vi "Main Test.vi"() -> ()   [LabVIEW 2021]
uses:
  Mete.ctl
  R.ctl
  P.ctl
  N.ctl
  D.ctl
  Odo Velocity.ctl
  Gas.ctl
  Set-.ctl
  Set+.ctl
  Cru.ctl
  Dis.ctl
panel:
  in  "Boolean 8":T1
  in  "Boolean 7":T2
  in  "Boolean 5":T3
  in  "Boolean 6":T4
  in  "Slide 2":T5
  out "Km/h":T6 scale=0.0..250.0
  in  "stop":bool
  in  "Slide":u32(slide) max=900 scale=0.0..999.0
  out "Boolean 4":T7
  out "Boolean 3":T8
  out "Boolean 2":T9
  out "Boolean":T10
  out "Gauge":T11 scale=0.0..650.0
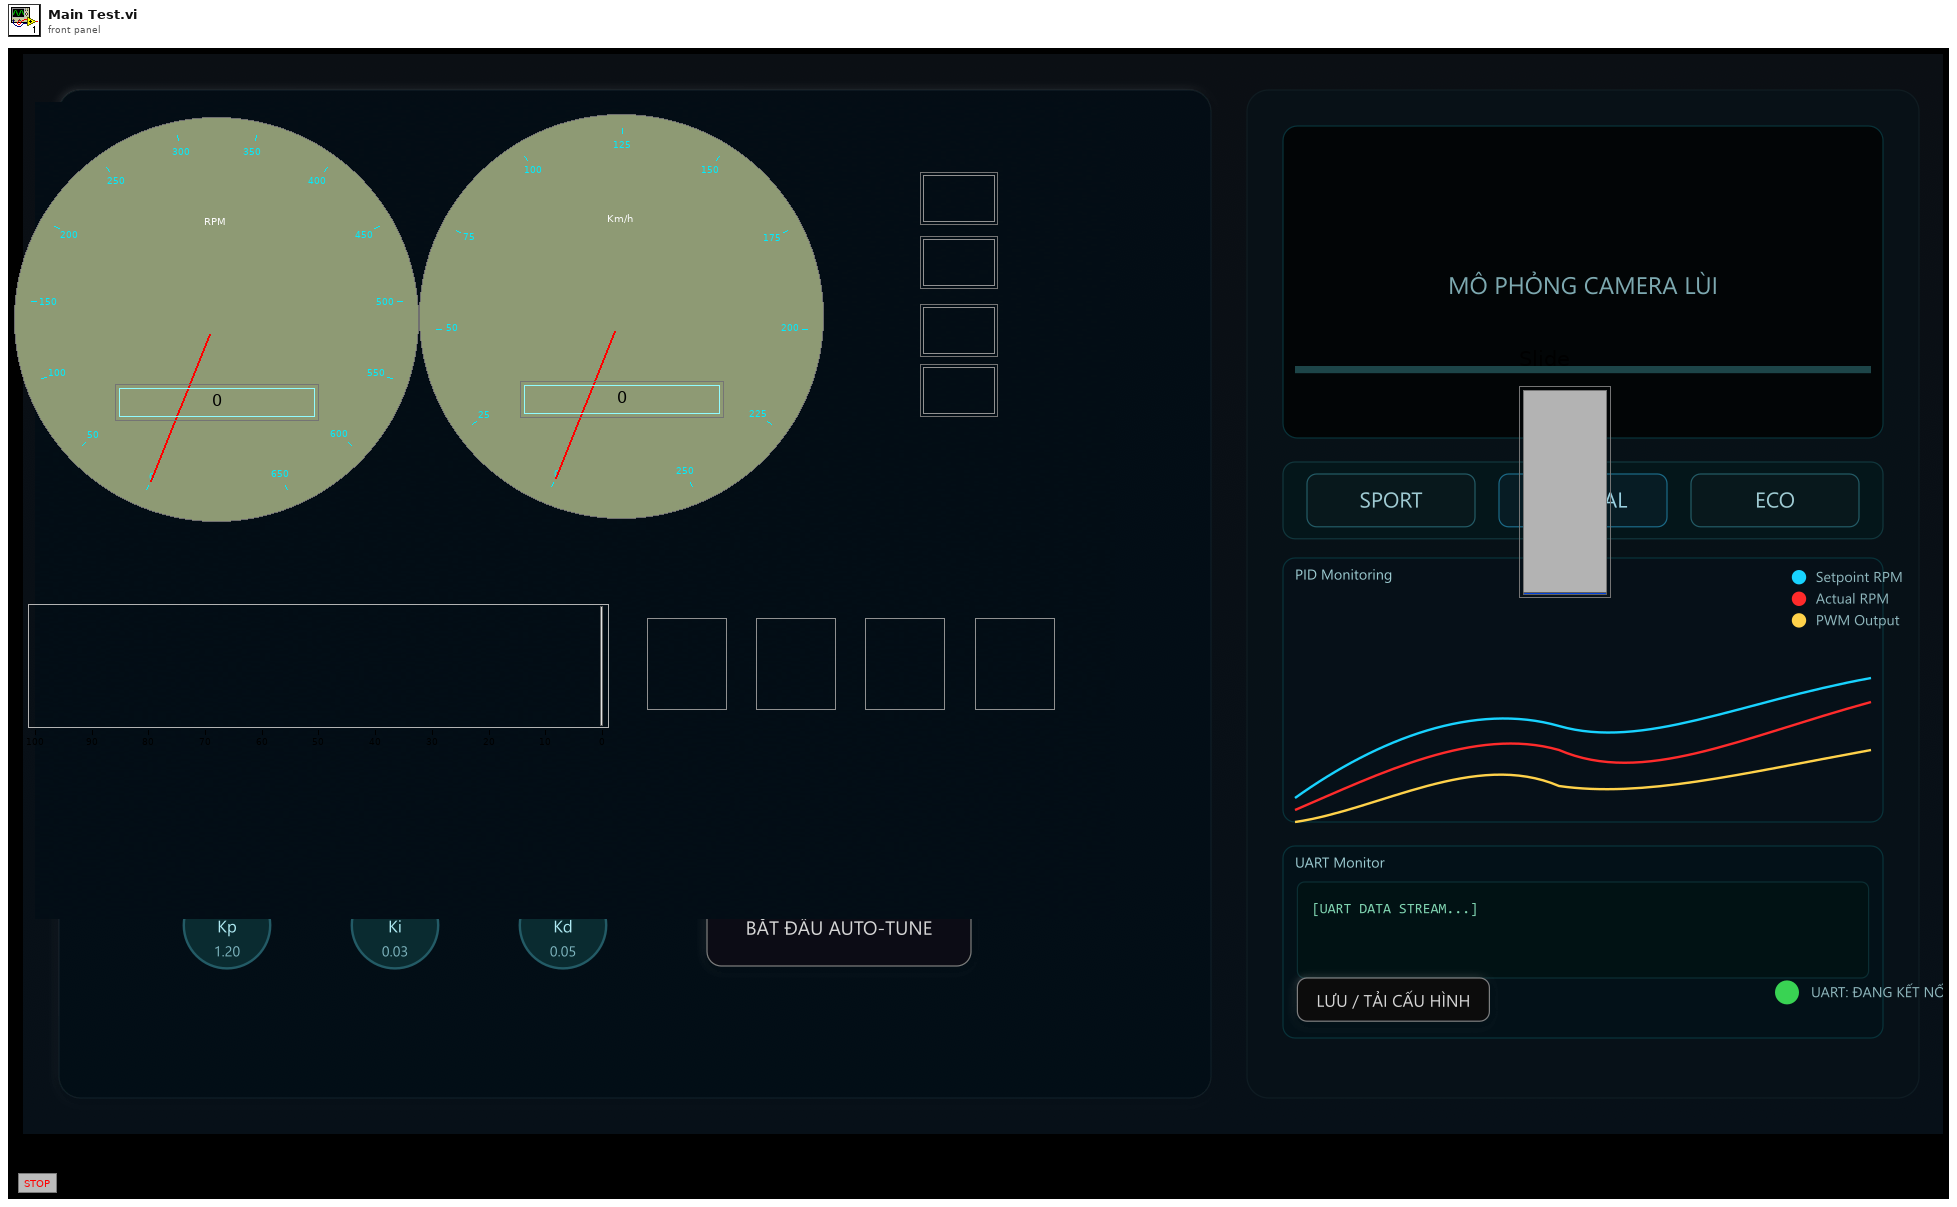
[diagram p1: front panel]
types:
  T1 = typedef "Dis.ctl" = bool
  T2 = typedef "Cru.ctl" = bool
  T3 = typedef "Set+.ctl" = bool
  T4 = typedef "Set-.ctl" = bool
  T5 = typedef "Gas.ctl" = dbl
  T6 = typedef "Odo Velocity.ctl" = u16
  T7 = typedef "D.ctl" = bool
  T8 = typedef "N.ctl" = bool
  T9 = typedef "P.ctl" = bool
  T10 = typedef "R.ctl" = bool
  T11 = typedef "Mete.ctl" = u16
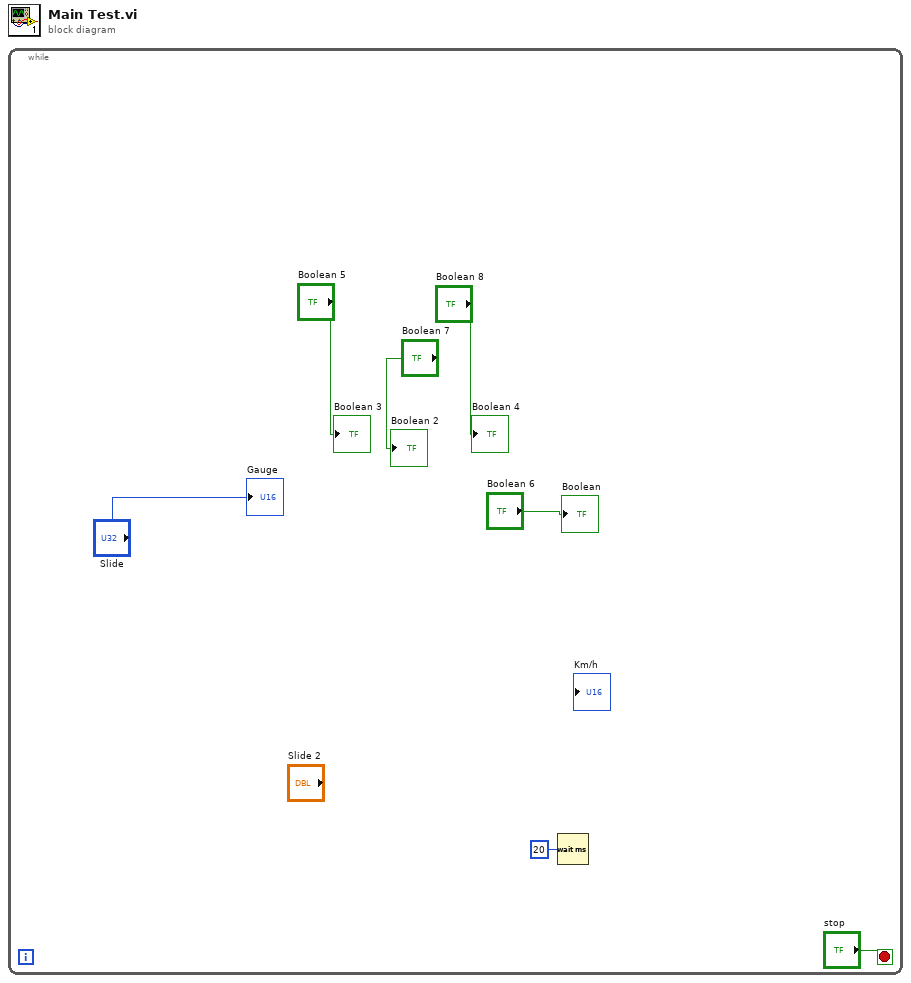
[diagram p0: block diagram]
diagram:
  n1 = while {
    stop <- "stop" stop-if-true
    n2 = Wait (ms)(milliseconds to wait=u32 20) -> ()  [unwired: 1 out]
    "Gauge" <- "Slide"
    "Boolean 2" <- "Boolean 7"
    "Boolean 3" <- "Boolean 5"
    "Boolean" <- "Boolean 6"
    "Boolean 4" <- "Boolean 8"
  }
